vi "round.vi"() -> ()   [LabVIEW 2019]
uses:
  subVI/move/move array.ctl
panel:
  out "Array":T1
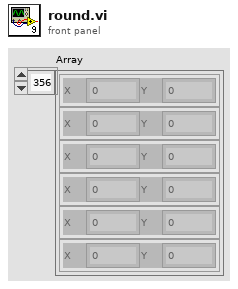
[diagram p1: front panel]
types:
  T1 = typedef "move array.ctl" = cluster{"X":dbl, "Y":dbl}[]
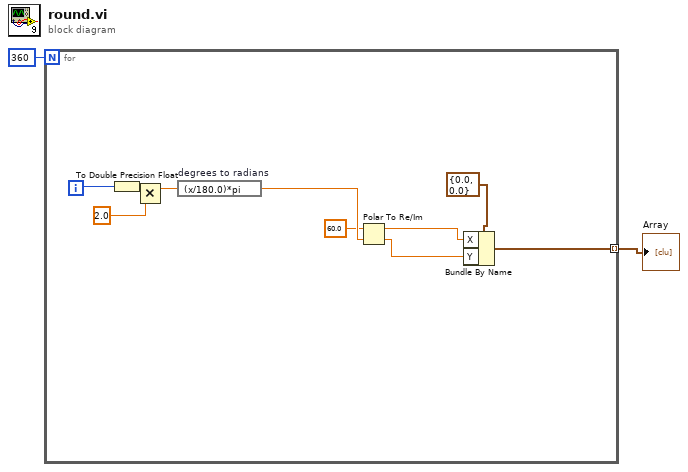
[diagram p0: block diagram]
diagram:
  n1 = for {
    N: 360 -> [_]
    tunnel: [w6] -> w1 mode=indexing
    i -> [w12]
    n2 = To Double Precision Float(number=w12) -> (double precision float=w11:dbl)
    n3 = Multiply(x=w11, y=2.0) -> (x*y=w4:dbl)
    n4 = expression code="(x/180.0)*pi" "degrees to radians"(w4) -> (w10:dbl)
    n5 = Polar To Re/Im(2:w10, 3:60.0 ("r")) -> (0:w7:dbl, 1:w8:dbl)
    n6 = Bundle By Name(cluster=cluster{"X":dbl, "Y":dbl} {"X"=0.0, "Y"=0.0} ("Cluster"), "X"=w8, "Y"=w7) -> (w6:cluster{"X":dbl, "Y":dbl})
  }
  "Array" <- w1
